vi "spectral_analysis.vi"(0 "Sampling frequency":dbl, 1 "Data":dbl format="%0.2f") -> (2 "Spectrum":dbl[](graph), 3 "?":i32(graph)=145, 5 "RMS":dbl(graph))   [LabVIEW 2023]
uses:
  <vilib>/ptbypt/NI_PtbyPt.lvlib
panel:
  out "Mean frequency":dbl=145.0
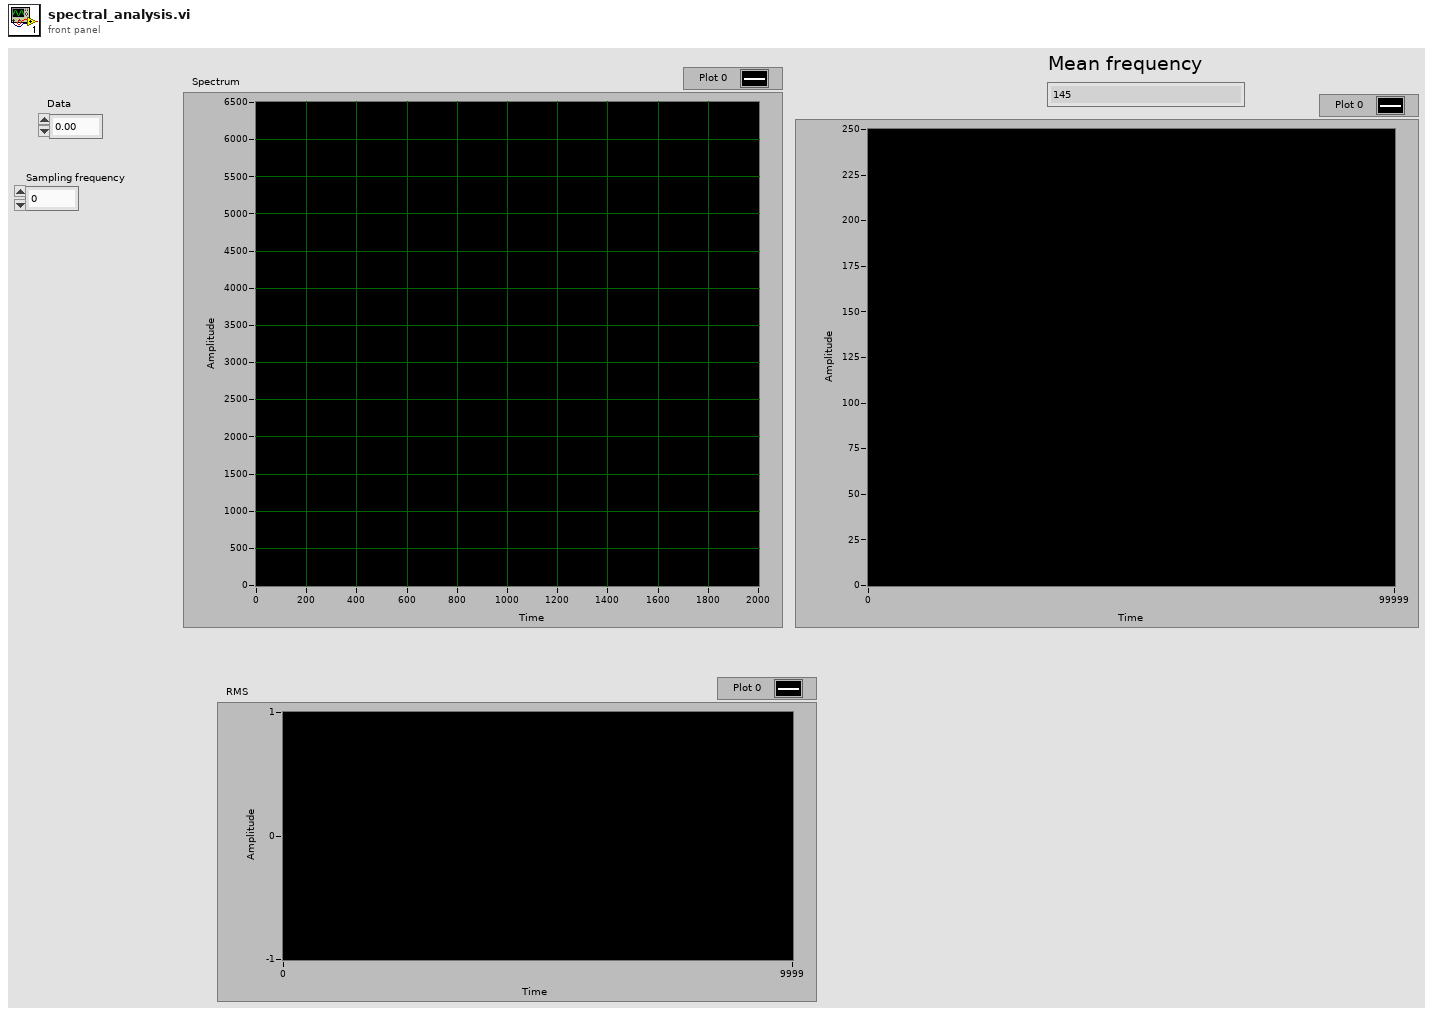
[diagram p1: front panel]
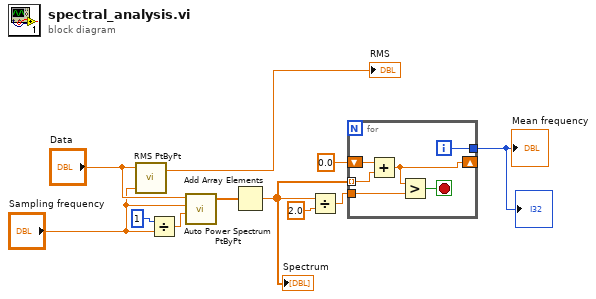
[diagram p0: block diagram]
diagram:
  n1 = call <vilib>:"RMS PtByPt.vi"("sample length"="Sampling frequency", "x"="Data") -> ("rms value"=→"RMS":dbl)  [unwired: 2 in, 1 out]
  n2 = Divide(x=1, y="Sampling frequency") -> (x/y=w4:dbl)
  n3 = call <vilib>:"Auto Power Spectrum PtByPt.vi"("signal"="Data", "sample length"="Sampling frequency", "dt"=w4) -> ("Power Spectrum (V^2 rms)"=w1:dbl[])  [unwired: 2 in, 2 out]
  "Spectrum" <- w1
  n4 = Add Array Elements(numeric array=w1) -> (sum=w11:dbl)
  n5 = Divide(x=w11, y=2.0) -> (x/y=w9:dbl)
  n6 = for {
    shift-right: [w15] -> _
    shift-left: 0.0 -> [w14]
    tunnel: w9 -> [w17]
    tunnel: w1 -> [w13] mode=indexing
    tunnel: [w12] -> w7
    i -> [w12]
    stop <- w16 stop-if-true
    n7 = Add(x=w14, y=w13) -> (x+y=w15:dbl)
    n8 = Greater?(x=w15, y=w17) -> (0:w16:bool)
  }
  "Mean frequency" <- w7
  "?" <- w7
